vi "Relay Test_TS.vi"(8 "error in (no error)":errorcluster, 10 "Message IN":string) -> (0 "error out":errorcluster, 1 "Result (bool)":bool, 2 "Message OUT":string, 3 "VISA resource name 2":refnum<visa-resource-name>)   [LabVIEW 2022 SP3]
uses:
  <vilib>/DAQmx/read.llb/DAQmx Read (Digital 1D Bool NChan 1Samp 1Line).vi
  <vilib>/DAQmx/miscellaneous.llb/DAQmx Fill In Error Info.vi
panel:
  out "Result (color)":u32(colorbox)
  out "cDAQ DI Reading":bool[](array[boolean])
  out "LC DO Cmd":bool[](array[boolean])
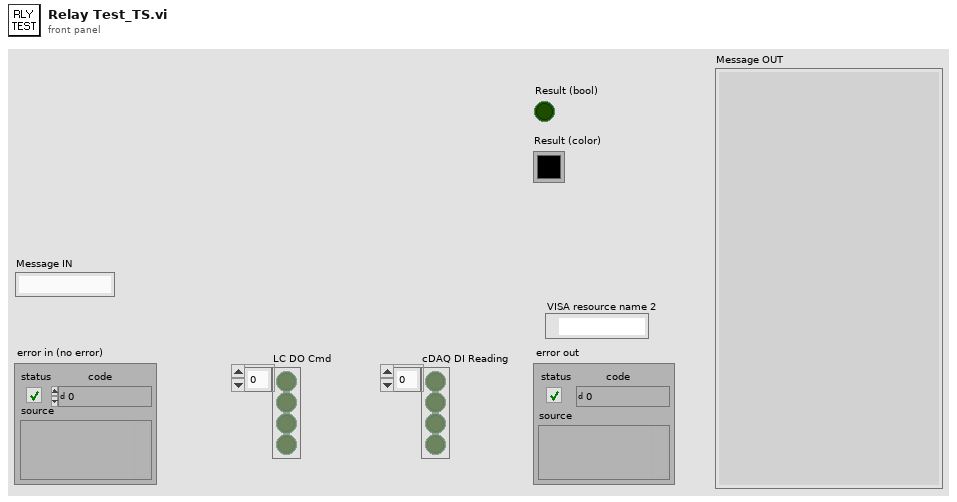
[diagram p1: front panel]
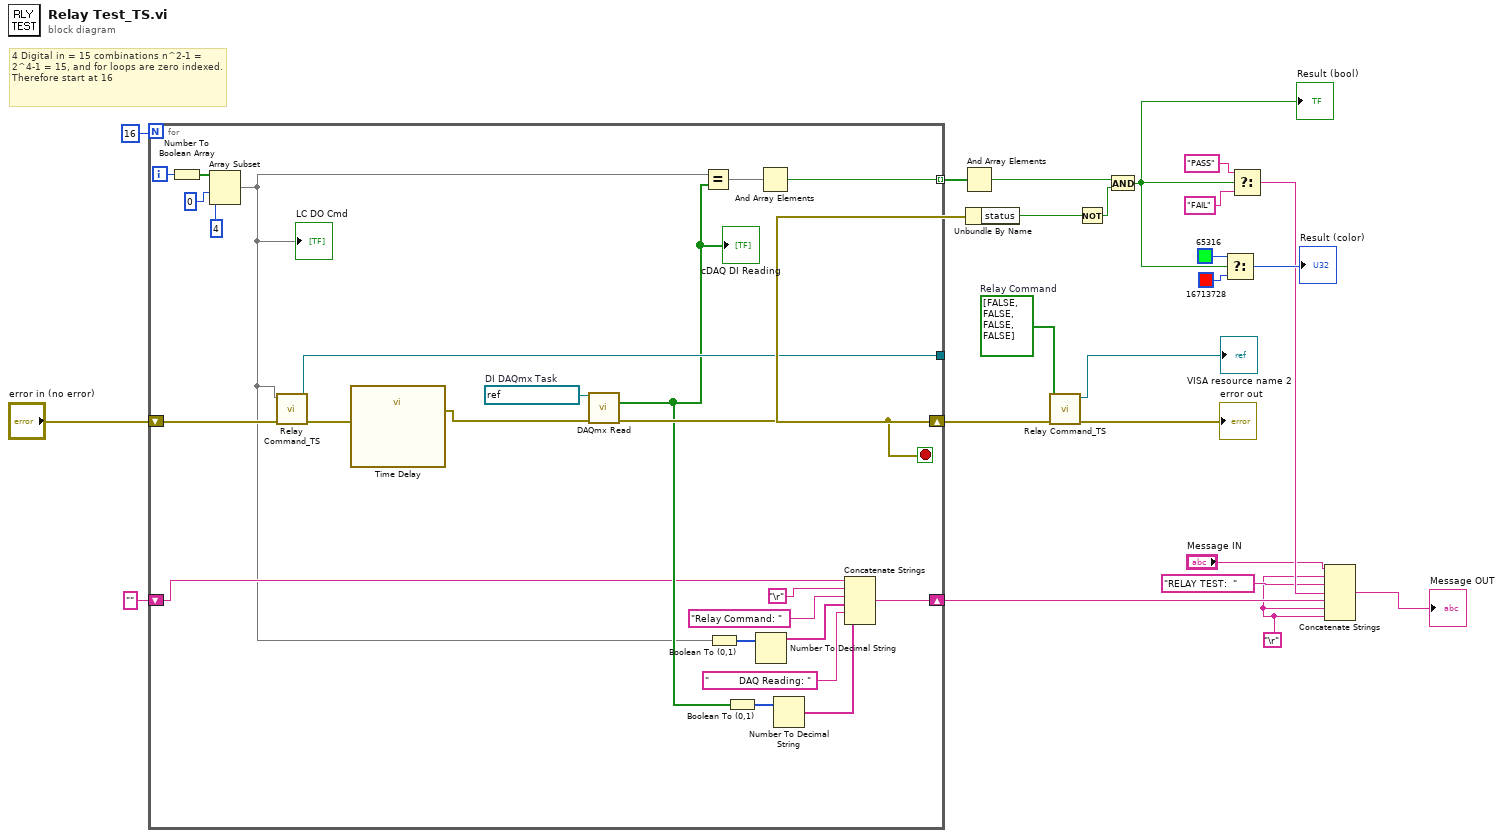
[diagram p0: block diagram]
diagram:
  w1 = bool[] [FALSE, FALSE, FALSE, FALSE]  # Relay Command
  w6 = "\r"
  # "4 Digital in = 15 combinations n^2-1 = 2^4-1 = 15, and for loops are zero indexed.  Therefore start at 16"
  n1 = for {
    N: 16 -> [_]
    shift-right: [w39] -> w4
    shift-left: "error in (no error)" -> [w44]
    tunnel: [w42] -> _
    tunnel: [w46] -> w23 mode=indexing
    shift-right: [w27] -> w10
    shift-left: "" -> [w26]
    i -> [w25]
    stop <- w39 stop-if-true
    w41 = refnum<k21> "FTS2_RelayIn"  # DI DAQmx Task
    n2 = Number To Boolean Array(number=w25) -> (Boolean array=w29:bool[])
    n3 = Array Subset(array=w29, index=0, length=4) -> (w24:bool[])
    "LC DO Cmd" <- w24
    n4 = call "Relay Command_TS.vi"("error in (no error)"=w44, "Relay Command"=w24) -> ("error out"=w43:errorcluster, "VISA Refnum out"=w42:refnum<visa-resource-name>)  [unwired: 8 in]
    n5 = call "Time Delay"("error in (no error)"=w43) -> ("error out"=w40:errorcluster)  [unwired: 10 in]
    n6 = call-poly <vilib>:"DAQmx Read.vi"("task/channels in"=w41, "error in"=w40) -> ("data"=w28:bool[], "error out"=w39:errorcluster)  [unwired: 11 in, 1 out]
    "cDAQ DI Reading" <- w28
    n7 = Equal?(x=w24, y=w28) -> (x = y?=w45:bool[])
    n8 = Boolean To (0,1)(Boolean=w24) -> (0, 1=w33:i16[])
    n9 = Boolean To (0,1)(Boolean=w28) -> (0, 1=w32:i16[])
    n10 = Number To Decimal String(number=w33) -> (decimal integer string=w36:string[])  [unwired: 1 in]
    n11 = And Array Elements(Boolean array=w45) -> (logical AND=w46:bool)
    n12 = Number To Decimal String(number=w32) -> (decimal integer string=w38:string[])  [unwired: 1 in]
    n13 = Concatenate Strings(w26, "\r", "Relay Command: ", w36, "          DAQ Reading: ", w38) -> (w27:string)
  }
  n14 = And Array Elements(Boolean array=w23) -> (logical AND=w12:bool)
  n15 = Unbundle By Name(w4) -> ("status"=w15:bool)
  n16 = call "Relay Command_TS.vi"("error in (no error)"=w4, "Relay Command"=w1) -> ("error out"=→"error out":errorcluster, "VISA Refnum out"=→"VISA resource name 2":refnum<visa-resource-name>)  [unwired: 8 in]
  n17 = Not(x=w15) -> (.not. x?=w14:bool)
  n18 = And(x=w12, y=w14) -> (x .and. y?=w13:bool)
  "Result (bool)" <- w13
  n19 = Select(t=u32 65316 ("Result (color)"), s=w13, f=u32 16713728 ("Result (color)")) -> (s? t:f=→"Result (color)":u32)
  n20 = Select(t="PASS", s=w13, f="FAIL") -> (s? t:f=w9:string)
  n21 = Concatenate Strings("Message IN", w6, "RELAY TEST:  ", w9, w10, w6, w6) -> (→"Message OUT":string)
